vi "Teleop.vi"(10 "Match Info":T1={"Autonomous Elapsed Seconds"=0.0, "TeleOp Elapsed Seconds"=0.0, "Disabled Elapsed Seconds"=0.0, "Visited Autonomous"=FALSE, "Visited TeleOp"=FALSE, "Visited Disabled"=FALSE, "Autonomous Settings"={"Autonomous Style"=enum."Independent", "VI Refnum"=refnum}}, 11 "Call Context":T2) -> ()   [LabVIEW 2017]
doc: "This VI is called for each TeleOp packet received from the DS where the robot is not disabled. It is often used to read from the joysticks and update I/O or to update setpoints for timed control loops. It should complete and return within 20 milliseconds or it may miss DS packets."
uses:
  <vilib>/Rock Robotics/WPI/DriverStation/WPI_DriverStationDerivedRobotMode.ctl
  <vilib>/Rock Robotics/WPI/DriverStation/WPI_DriverStationMatch Info.ctl
  <vilib>/Rock Robotics/WPI/Utilities/WPI_GetSetVariantRefNum.vi
  <vilib>/Rock Robotics/Network Tables/NT Write Boolean Array.vi
  <vilib>/Rock Robotics/Network Tables/NT Write Numeric Array.vi
  <vilib>/Rock Robotics/Network Tables/NT Read Boolean.vi
  <vilib>/Rock Robotics/Network Tables/NT Read Number.vi
panel:
  out "Sample Slider 0":dbl(slide) scale=0.0..5.0
  out "Sample Boolean 1":bool
  out "Sample Boolean 0":bool
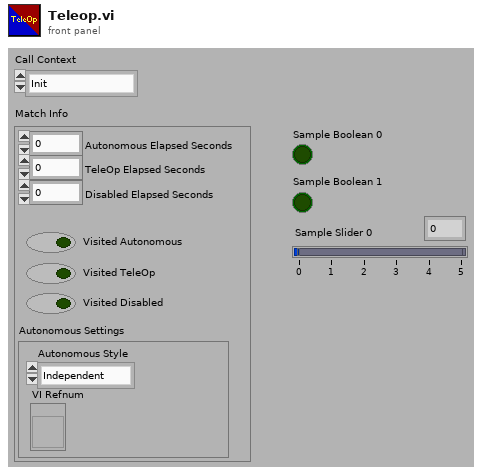
[diagram p1: front panel]
types:
  T1 = typedef "WPI_DriverStationMatch Info.ctl" = cluster{"Autonomous Elapsed Seconds":dbl, "TeleOp Elapsed Seconds":dbl, "Disabled Elapsed Seconds":dbl, "Visited Autonomous":bool, "Visited TeleOp":bool, "Visited Disabled":bool, "Autonomous Settings":cluster{"Autonomous Style":enum16{"Iterative", "Independent"}, "VI Refnum":refnum<vi>}}
  T2 = typedef "WPI_DriverStationDerivedRobotMode.ctl" = enum16{"Init", "Execute", "Stop"}
  T3 = typedef "WPI_RobotDriveDevRef.ctl" = cluster{"DevStatus":errorcluster, "Motors[]":T4[], "Square Inputs":bool, "Max Output":dbl}
  T4 = typedef "WPI_MotorControlDeviceRef.ctl" = cluster{"DeviceStatus":errorcluster, "Type":T5, "PWM":cluster{"PWM Channel":T6, "DeadBand":T7}, "CAN":cluster{"Device Number":u8, "SetOutput VI Ref":variant, "GetOutput VI Ref":variant, "Enable VI Ref":variant, "Disable VI Ref":variant, "Data":variant}, "Invert":bool, "DIO PWM":cluster{"PWM \"Enable\" Channel":T6, "DIOChannel":T8, "PWM Rate":dbl}}
  T5 = typedef "WPI_MotorControlType.ctl" = enum16{"PWM", "CAN", "DIO PWM"}
  T6 = typedef "FPGA_DIOPWMChannel.ctl" = enum8{"PWM 0", "PWM 1", "PWM 2", "PWM 3", "PWM 4", "PWM 5", "PWM 6", "PWM 7", "PWM 8", "PWM 9", "PWM MXP 0", "PWM MXP 1", "PWM MXP 2", "PWM MXP 3", "PWM MXP 4", "PWM MXP 5", "PWM MXP 6", "PWM MXP 7", "PWM MXP 8", "PWM MXP 9", "Invalid"}
  T7 = typedef "WPI_PWMDeadband.ctl" = cluster{"Name":string, "maxPositivePwm":i32, "minPositivePwm":i32, "centerPwm":i32, "maxNegativePwm":i32, "minNegativePwm":i32, "angularRange":u16}
  T8 = typedef "FPGA_DIOChannel.ctl" = enum8{"DIO 0", "DIO 1", "DIO 2", "DIO 3", "DIO 4", "DIO 5", "DIO 6", "DIO 7", "DIO 8", "DIO 9", "DIO MXP 0", "DIO MXP 1", "DIO MXP 2", "DIO MXP 3", "DIO MXP 4", "DIO MXP 5", "DIO MXP 6", "DIO MXP 7", "DIO MXP 8", "DIO MXP 9", "DIO MXP 10", "DIO MXP 11", "DIO MXP 12", "DIO MXP 13", "DIO MXP 14", "DIO MXP 15", "SPI Port CS1", "SPI Port CS2", "SPI Port CS3", "SPI Port MISO", "SPI Port MOSI", "Invalid"}
  T9 = typedef "WPI_JoystickDevRef.ctl" = cluster{"Device":T10}
  T10 = typedef "WPI_JoystickDeviceEnum.ctl" = enum16{"USB 0", "USB 1", "USB 2", "USB 3", "USB 4", "USB 5"}
  T11 = typedef "WPI_SwitchDevRef.ctl" = cluster{"DevStatus":errorcluster, "DIO Channel":T8, "CntIndex":T12, "Normally Closed":bool}
  T12 = typedef "FPGA_CounterCtrSystemIndex.ctl" = enum8{"Ctr 0", "Ctr 1", "Ctr 2", "Ctr 3", "Ctr 4", "Ctr 5", "Ctr 6", "Ctr 7", "Invalid"}
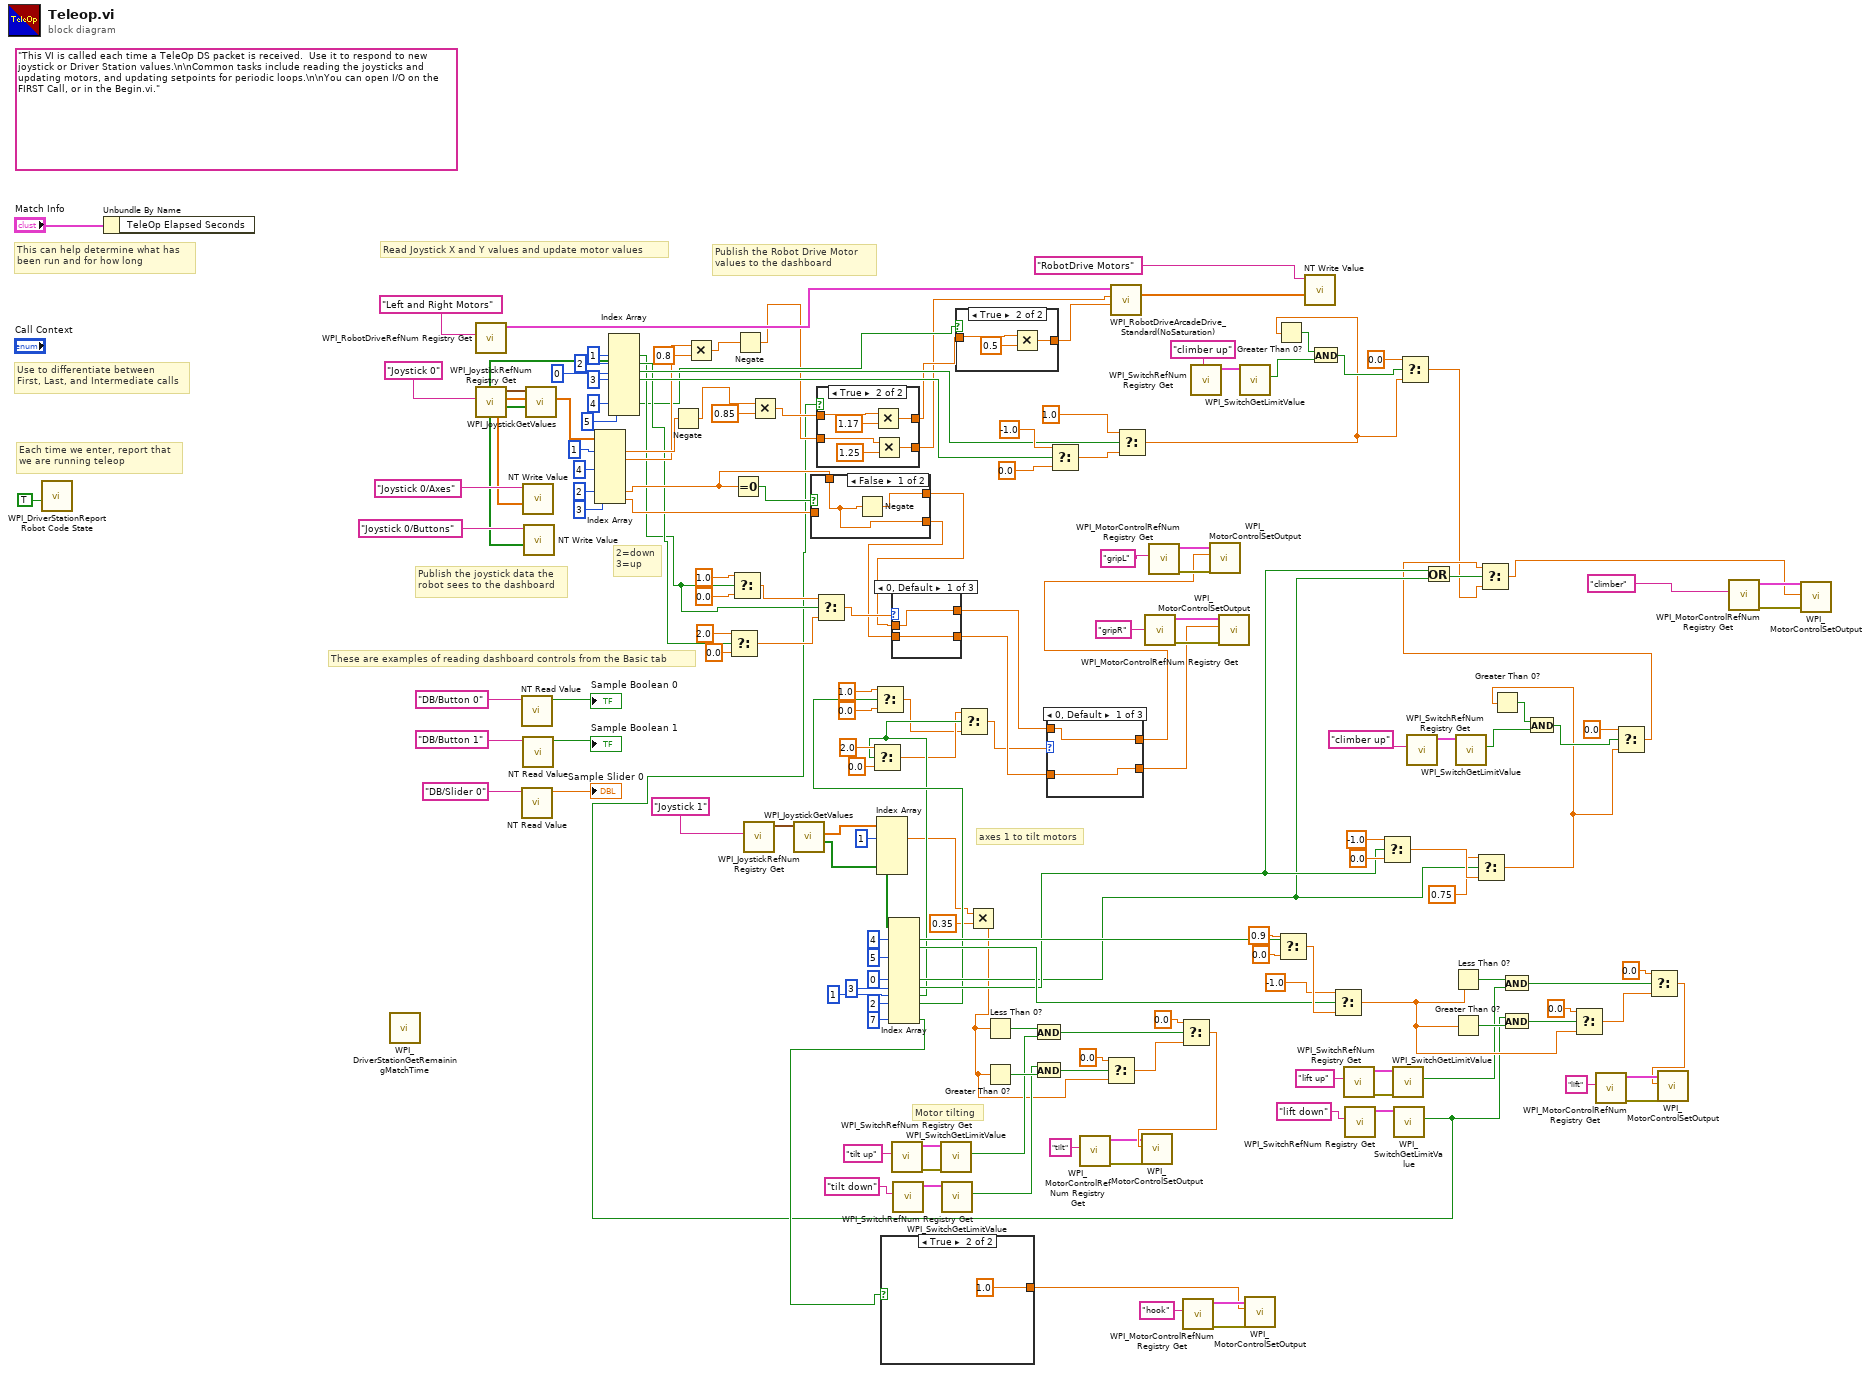
[diagram p0: block diagram]
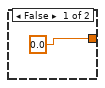
[diagram p2: hidden frame]
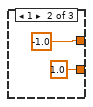
[diagram p5: hidden frame]
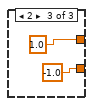
[diagram p6: hidden frame]
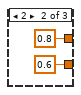
[diagram p7: hidden frame]
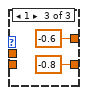
[diagram p8: hidden frame]
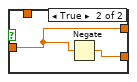
[diagram p9: hidden frame]
diagram:
  (unwired) "This VI is called each time a TeleOp DS packet is received.  Use it to respond to new joystick or Driver Station values.\n\nCommon tasks include reading the joysticks and updating motors, and updating setpoints for periodic loops.\n\nYou can open I/O on the FIRST Call, or in the Begin.vi."
  # "Motor tilting"
  # "axes 1 to tilt motors"
  # "2=down\n3=up"
  # "These are examples of reading dashboard controls from the Basic tab"
  # "Publish the Robot Drive Motor\nvalues to the dashboard"
  # "Publish the joystick data the\nrobot sees to the dashboard"
  # "Each time we enter, report that\nwe are running teleop"
  # "Use to differentiate between\nFirst, Last, and Intermediate calls"
  # "This can help determine what has\nbeen run and for how long"
  # "Read Joystick X and Y values and update motor values"
  n1 = call <vilib>:"WPI_DriverStationReport Robot Code State.vi"("TeleOp"=TRUE ("Autonomous")) -> ()  [unwired: 10 in, 1 out]
  n2 = Unbundle By Name("Match Info") -> ()  [unwired: 1 out]
  n3 = call <vilib>:"WPI_DriverStationGetRemainingMatchTime.vi"() -> ()  [unwired: 10 in, 2 out]
  n4 = call <vilib>:"WPI_RobotDriveRefNum Registry Get.vi"("refnum name"="Left and Right Motors") -> ("RobotDriveDevRef"=w167:T3)  [unwired: 1 in, 9 out]
  n5 = call <vilib>:"WPI_JoystickRefNum Registry Get.vi"("refnum name"="Joystick 0") -> ("JoystickDevRef"=w165:T9)  [unwired: 1 in, 9 out]
  n6 = call-poly <vilib>:"NT Read Value.vi"("Name"="DB/Button 0" ("refnum name")) -> ("Boolean"=→"Sample Boolean 0":bool)  [unwired: 9 in, 1 out]
  n7 = call-poly <vilib>:"NT Read Value.vi"("Name"="DB/Slider 0" ("refnum name")) -> ("Numeric"=→"Sample Slider 0":dbl)  [unwired: 9 in, 1 out]
  n8 = call-poly <vilib>:"NT Read Value.vi"("Name"="DB/Button 1" ("refnum name")) -> ("Boolean"=→"Sample Boolean 1":bool)  [unwired: 9 in, 1 out]
  n9 = call <vilib>:"WPI_JoystickGetValues.vi"("JoystickDevRef"=w165) -> ("Buttons"=w148:bool[], "Axes"=w161:dbl[])  [unwired: 6 in, 3 out]
  n10 = call-poly <vilib>:"NT Write Value.vi"("Numeric Array"=w161, "Name"="Joystick 0/Axes") -> ()  [unwired: 9 in, 1 out]
  n11 = call-poly <vilib>:"NT Write Value.vi"("Boolean Array"=w148, "Name"="Joystick 0/Buttons") -> ()  [unwired: 9 in, 1 out]
  n12 = Index Array(array=w161, index #1=1 ("index"), index #2=4 ("index"), index #6=2 ("index"), index #7=3 ("index")) -> (element #1=w135:dbl, element #2=w126:dbl, element #6=w129:dbl, element #7=w130:dbl)  [unwired: 3 in, 3 out]
  n13 = Index Array(array=w148, index #1=1 ("index"), index #2=2 ("index"), index #3=0 ("index"), index #4=3 ("index"), index #7=4 ("index"), index #8=5 ("index")) -> (element #1=w56:bool, element #2=w59:bool, element #3=w136:bool, element #4=w143:bool, element #7=w42:bool)  [unwired: 2 in, 3 out]
  n14 = Negate(x=w135) -> (-x=w128:dbl)
  n15 = Multiply(x=w126, y=0.8) -> (x*y=w124:dbl)
  n16 = Select(t=2.0, s=w59, f=0.0) -> (s? t:f=w60:dbl)
  n17 = Select(t=1.0, s=w56, f=0.0) -> (s? t:f=w61:dbl)
  n18 = Equal To 0?(x=w129) -> (x = 0?=w131:bool)
  n19 = Negate(x=w124) -> (-x=w41:dbl)
  n20 = call <vilib>:"WPI_JoystickRefNum Registry Get.vi"("refnum name"="Joystick 1") -> ("JoystickDevRef"=w151:T9)  [unwired: 1 in, 9 out]
  n21 = Multiply(x=w128, y=0.85) -> (x*y=w45:dbl)
  n22 = call <vilib>:"WPI_JoystickGetValues.vi"("JoystickDevRef"=w151) -> ("Buttons"=w95:bool[], "Axes"=w150:dbl[])  [unwired: 6 in, 3 out]
  n23 = case shown="False" w131 {
    tunnel: [w171 w173] -> w54
    tunnel: w130 -> [_ w173]
    tunnel: w129 -> [w170 _]
    tunnel: [w170 w172] -> w53
    frame False {
      n24 = Negate(x=w170) -> (-x=w171:dbl)
    }
    frame True {
      n25 = Negate(x=w173) -> (-x=w172:dbl)
    }
  }
  n26 = Select(t=w61, s=w56, f=w60) -> (s? t:f=w55:dbl)
  n27 = Index Array(array=w150, index #1=1 ("index")) -> (element #1=w4:dbl)  [unwired: 4 in, 4 out]
  n28 = Index Array(array=w95, index #1=4 ("index"), index #2=5 ("index"), index #6=0 ("index"), index #7=3 ("index"), index #8=1 ("index"), index #9=2 ("index"), index #11=7 ("index")) -> (element #1=w92:bool, element #2=w91:bool, element #6=w72:bool, element #7=w73:bool, element #8=w33:bool, element #9=w34:bool, element #11=w6:bool)  [unwired: 4 in, 4 out]
  n29 = Select(t=2.0, s=w33, f=0.0) -> (s? t:f=w12:dbl)
  n30 = Select(t=1.0, s=w34, f=0.0) -> (s? t:f=w11:dbl)
  n31 = case shown="True" w6 {
    tunnel: [0.0 ("Output") 1.0 ("Output")] -> w5
    frame False {
    }
    frame True {
    }
  }
  n32 = case shown="0, Default" w55 {
    tunnel: [w177 0.8 ("upper limit") -0.6 ("upper limit")] -> w50
    tunnel: w54 -> [w177 _ _]
    tunnel: [w176 0.6 ("upper limit") -0.8 ("upper limit")] -> w48
    tunnel: w53 -> [w176 _ _]
    frame 0, Default {
    }
    frame 2 {
    }
    frame 1 {
    }
  }
  n33 = call <vilib>:"WPI_SwitchRefNum Registry Get.vi"("refnum name"="tilt up") -> ("error out"=w30:errorcluster, "SwitchDevRef"=w29:T11)  [unwired: 9 in]
  n34 = call <vilib>:"WPI_SwitchRefNum Registry Get.vi"("refnum name"="tilt down") -> ("SwitchDevRef"=w28:T11)  [unwired: 9 in, 1 out]
  n35 = call <vilib>:"WPI_SwitchGetLimitValue.vi"("error in (no error)"=w30, "SwitchDevRef"=w29) -> ("Switch Pressed"=w15:bool)  [unwired: 7 in, 2 out]
  n36 = call <vilib>:"WPI_SwitchGetLimitValue.vi"("SwitchDevRef"=w28) -> ("Switch Pressed"=w16:bool)  [unwired: 8 in, 2 out]
  n37 = Select(t=w12, s=w33, f=w11) -> (s? t:f=w32:dbl)
  n38 = Multiply(x=w4, y=0.35) -> (x*y=w3:dbl)
  n39 = Less Than 0?(x=w3) -> (x < 0?=w20:bool)
  n40 = Greater Than 0?(x=w3) -> (x > 0?=w21:bool)
  n41 = And(x=w20, y=w15) -> (x .and. y?=w22:bool)
  n42 = And(x=w16, y=w21) -> (x .and. y?=w23:bool)
  n43 = case shown="0, Default" w32 {
    tunnel: [w182 -1.0 ("upper limit") 1.0 ("upper limit")] -> w51
    tunnel: w50 -> [w182 _ _]
    tunnel: [w183 1.0 ("upper limit") -1.0 ("upper limit")] -> w49
    tunnel: w48 -> [w183 _ _]
    frame 0, Default {
    }
    frame 1 {
    }
    frame 2 {
    }
  }
  n44 = Select(t=-1.0, s=w143, f=0.0) -> (s? t:f=w140:dbl)
  n45 = call <vilib>:"WPI_MotorControlRefNum Registry Get.vi"("refnum name"="tilt") -> ("error out"=w24:errorcluster, "MotorControlDevRef"=w13:T4)  [unwired: 9 in]
  n46 = Select(t=0.0, s=w23, f=w3) -> (s? t:f=w17:dbl)
  n47 = Select(t=1.0, s=w136, f=w140) -> (s? t:f=w117:dbl)
  n48 = call <vilib>:"WPI_MotorControlRefNum Registry Get.vi"("refnum name"="gripR") -> ("error out"=w67:errorcluster, "MotorControlDevRef"=w47:T4)  [unwired: 9 in]
  n49 = call <vilib>:"WPI_MotorControlRefNum Registry Get.vi"("refnum name"="gripL") -> ("error out"=w132:errorcluster, "MotorControlDevRef"=w133:T4)  [unwired: 9 in]
  n50 = Select(t=0.0, s=w22, f=w17) -> (s? t:f=w14:dbl)
  n51 = call <vilib>:"WPI_MotorControlSetOutput.vi"("error in (no error)"=w24, "Output"=w14, "MotorControlDevRef"=w13) -> ()  [unwired: 6 in, 3 out]
  n52 = call <vilib>:"WPI_MotorControlRefNum Registry Get.vi"("refnum name"="hook") -> ("error out"=w9:errorcluster, "MotorControlDevRef"=w8:T4)  [unwired: 9 in]
  n53 = call <vilib>:"WPI_SwitchRefNum Registry Get.vi"("refnum name"="climber up") -> ("SwitchDevRef"=w123:T11)  [unwired: 9 in, 1 out]
  n54 = call <vilib>:"WPI_MotorControlSetOutput.vi"("error in (no error)"=w132, "Output"=w51, "MotorControlDevRef"=w133) -> ()  [unwired: 6 in, 3 out]
  n55 = call <vilib>:"WPI_MotorControlSetOutput.vi"("error in (no error)"=w67, "Output"=w49, "MotorControlDevRef"=w47) -> ()  [unwired: 6 in, 3 out]
  n56 = call <vilib>:"WPI_SwitchGetLimitValue.vi"("SwitchDevRef"=w123) -> ("Switch Pressed"=w121:bool)  [unwired: 8 in, 2 out]
  n57 = call <vilib>:"WPI_MotorControlSetOutput.vi"("error in (no error)"=w9, "Output"=w5, "MotorControlDevRef"=w8) -> ()  [unwired: 6 in, 3 out]
  n58 = Greater Than 0?(x=w117) -> (x > 0?=w120:bool)
  n59 = Select(t=0.9, s=w92, f=0.0) -> (s? t:f=w111:dbl)
  n60 = And(x=w120, y=w121) -> (x .and. y?=w118:bool)
  n61 = Select(t=-1.0, s=w91, f=w111) -> (s? t:f=w102:dbl)
  n62 = call <vilib>:"WPI_SwitchRefNum Registry Get.vi"("refnum name"="lift up") -> ("error out"=w100:errorcluster, "SwitchDevRef"=w99:T11)  [unwired: 9 in]
  n63 = call <vilib>:"WPI_SwitchRefNum Registry Get.vi"("refnum name"="lift down") -> ("SwitchDevRef"=w98:T11)  [unwired: 9 in, 1 out]
  n64 = Select(t=-1.0, s=w73, f=0.0) -> (s? t:f=w85:dbl)
  n65 = call <vilib>:"WPI_SwitchGetLimitValue.vi"("error in (no error)"=w100, "SwitchDevRef"=w99) -> ("Switch Pressed"=w96:bool)  [unwired: 7 in, 2 out]
  n66 = call <vilib>:"WPI_SwitchGetLimitValue.vi"("SwitchDevRef"=w98) -> ("Switch Pressed"=w1:bool)  [unwired: 8 in, 2 out]
  n67 = case shown="True" w1 {
    tunnel: w45 -> [w189 w195]
    tunnel: [w189 w193] -> w44
    tunnel: w41 -> [w188 w191]
    tunnel: [w188 w190] -> w40
    frame False {
    }
    frame True {
      n68 = Multiply(x=w195, y=1.17) -> (x*y=w193:dbl)
      n69 = Multiply(x=w191, y=1.25) -> (x*y=w190:dbl)
    }
  }
  n70 = case shown="True" w42 {
    tunnel: w44 -> [w196 w199]
    tunnel: [w196 w197] -> w43
    frame False {
    }
    frame True {
      n71 = Multiply(x=w199, y=0.5) -> (x*y=w197:dbl)
    }
  }
  n72 = call <vilib>:"WPI_RobotDriveArcadeDrive_Standard(NoSaturation).vi"("Y axis value"=w43, "X axis value"=w40, "RobotDriveDevRef"=w167) -> ("Motor Values"=w154:dbl[])  [unwired: 1 in, 7 out]
  n73 = call-poly <vilib>:"NT Write Value.vi"("Numeric Array"=w154, "Name"="RobotDrive Motors") -> ()  [unwired: 9 in, 1 out]
  n74 = Select(t=0.0, s=w118, f=w117) -> (s? t:f=w69:dbl)
  n75 = call <vilib>:"WPI_SwitchRefNum Registry Get.vi"("refnum name"="climber up") -> ("SwitchDevRef"=w83:T11)  [unwired: 9 in, 1 out]
  n76 = Or(x=w73, y=w72) -> (x .or. y?=w71:bool)
  n77 = Less Than 0?(x=w102) -> (x < 0?=w106:bool)
  n78 = Greater Than 0?(x=w102) -> (x > 0?=w107:bool)
  n79 = call <vilib>:"WPI_SwitchGetLimitValue.vi"("SwitchDevRef"=w83) -> ("Switch Pressed"=w81:bool)  [unwired: 8 in, 2 out]
  n80 = Select(t=0.75, s=w72, f=w85) -> (s? t:f=w77:dbl)
  n81 = Greater Than 0?(x=w77) -> (x > 0?=w80:bool)
  n82 = And(x=w106, y=w96) -> (x .and. y?=w108:bool)
  n83 = And(x=w1, y=w107) -> (x .and. y?=w109:bool)
  n84 = And(x=w80, y=w81) -> (x .and. y?=w78:bool)
  n85 = Select(t=0.0, s=w109, f=w102) -> (s? t:f=w103:dbl)
  n86 = call <vilib>:"WPI_MotorControlRefNum Registry Get.vi"("refnum name"="lift") -> ("error out"=w114:errorcluster, "MotorControlDevRef"=w115:T4)  [unwired: 9 in]
  n87 = Select(t=0.0, s=w78, f=w77) -> (s? t:f=w70:dbl)
  n88 = Select(t=w70, s=w71, f=w69) -> (s? t:f=w68:dbl)
  n89 = Select(t=0.0, s=w108, f=w103) -> (s? t:f=w101:dbl)
  n90 = call <vilib>:"WPI_MotorControlSetOutput.vi"("error in (no error)"=w114, "Output"=w101, "MotorControlDevRef"=w115) -> ()  [unwired: 6 in, 3 out]
  n91 = call <vilib>:"WPI_MotorControlRefNum Registry Get.vi"("refnum name"="climber") -> ("error out"=w88:errorcluster, "MotorControlDevRef"=w89:T4)  [unwired: 9 in]
  n92 = call <vilib>:"WPI_MotorControlSetOutput.vi"("error in (no error)"=w88, "Output"=w68, "MotorControlDevRef"=w89) -> ()  [unwired: 6 in, 3 out]
